vi "Tools_Windows CPU Usage Close.vi"(8 "error in":errorcluster, 11 "CPU Usage Ref":T1) -> (0 "error out":errorcluster)   [LabVIEW 2014]
doc: "Unload the CPU Usage monitoring function."
uses:
  Windows/System32/pdh.dll
  tools_windows CPU Usage Ref.ctl
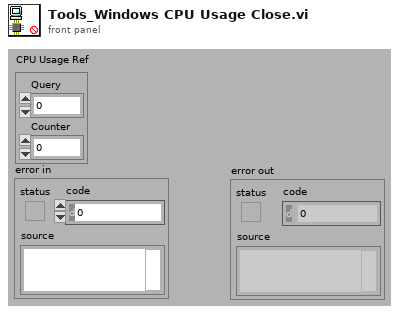
[diagram p1: front panel]
types:
  T1 = typedef "tools_windows CPU Usage Ref.ctl" = cluster{"Query":u32, "Counter":u32}
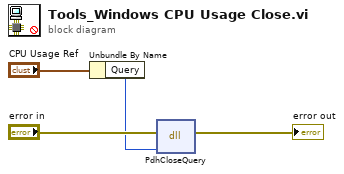
[diagram p0: block diagram]
diagram:
  n1 = Unbundle By Name("CPU Usage Ref") -> ("Query"=w1:u32)
  n2 = dll-call lib="/////Windows/System32/pdh.dll" fn="PdhCloseQuery"(error in="error in", "hQuery"=w1) -> (error out=→"error out":errorcluster)  [unwired: 4 in, 1 out]
